vi "2DStatistics.vi"(10 "data":u16[][](array[numeric])) -> (2 "Average":dbl, 3 "StDev":dbl)   [LabVIEW 2014]
uses:
  <vilib>/Analysis/NI_AALBase.lvlib
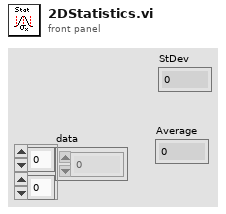
[diagram p1: front panel]
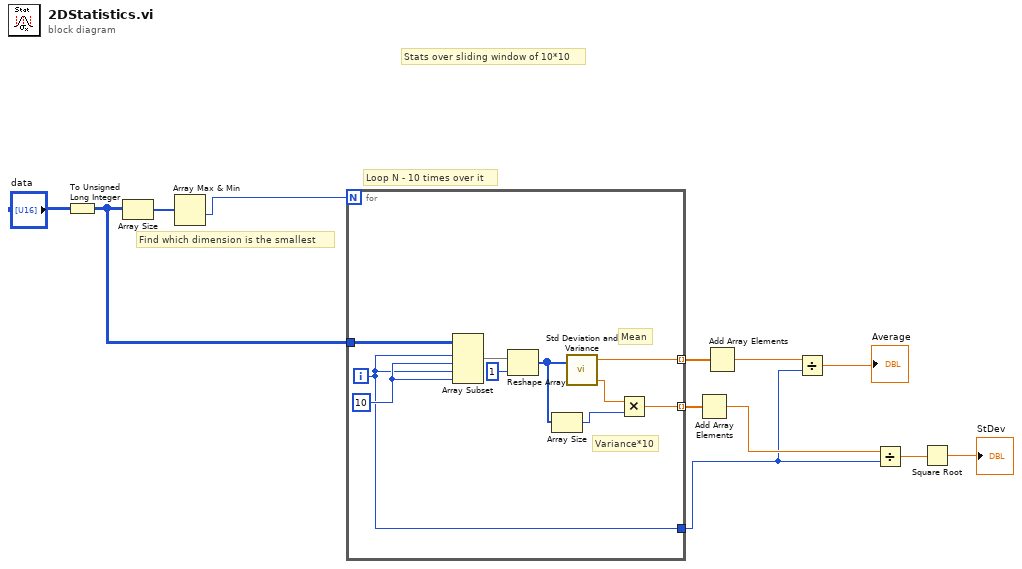
[diagram p0: block diagram]
diagram:
  # "Loop N - 10 times over it"
  # "Stats over sliding window of 10*10"
  # "Find which dimension is the smallest"
  n1 = To Unsigned Long Integer(number="data") -> (unsigned 32bit integer=w9:u32[][])
  n2 = Array Size(array=w9) -> (size(s)=w11:i32[])
  n3 = Array Max & Min(array=w11) -> (min value=w10:i32)  [unwired: 3 out]
  n4 = for {
    N: w10 -> [_]
    tunnel: w9 -> [w22]
    tunnel: [w18] -> w6 mode=indexing
    tunnel: [w14] -> w8 mode=indexing
    tunnel: [w13] -> w4
    i -> [w13]
    w21 = 10
    # "Mean"
    # "Variance*10"
    n5 = Array Subset(array=w22, index (row)=w13, length (row)=w21, index (col)=w13, length (col)=w21) -> (w20:u32[][])
    n6 = Reshape Array(w20, 1 ("dimension size")) -> (w17:u32[])
    n7 = Array Size(array=w17) -> (size(s)=w15:i32)
    n8 = call <vilib>:"Std Deviation and Variance.vi"("X"=w17) -> ("mean"=w18:dbl, "variance"=w16:dbl)  [unwired: 1 in, 1 out]
    n9 = Multiply(x=w16, y=w15) -> (x*y=w14:dbl)
  }
  n10 = Add Array Elements(numeric array=w8) -> (sum=w7:dbl)
  n11 = Add Array Elements(numeric array=w6) -> (sum=w5:dbl)
  n12 = Divide(x=w5, y=w4) -> (x/y=→"Average":dbl)
  n13 = Divide(x=w7, y=w4) -> (x/y=w2:dbl)
  n14 = Square Root(x=w2) -> (sqrt(x)=→"StDev":dbl)
